vi "TEST - Trim Whitespace (Performance).vi"() -> ()   [LabVIEW 2009]
uses:
  source/library/Trim Whitespace/Trim Whitespace (String).vi
  source/library/Trim Whitespace 1/Trim Whitespace (String) 1.vi
panel:
  out "Time New (ms)":u32
  out "Time Old (ms)":u32
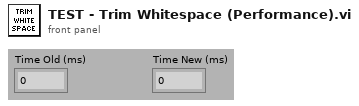
[diagram p1: front panel]
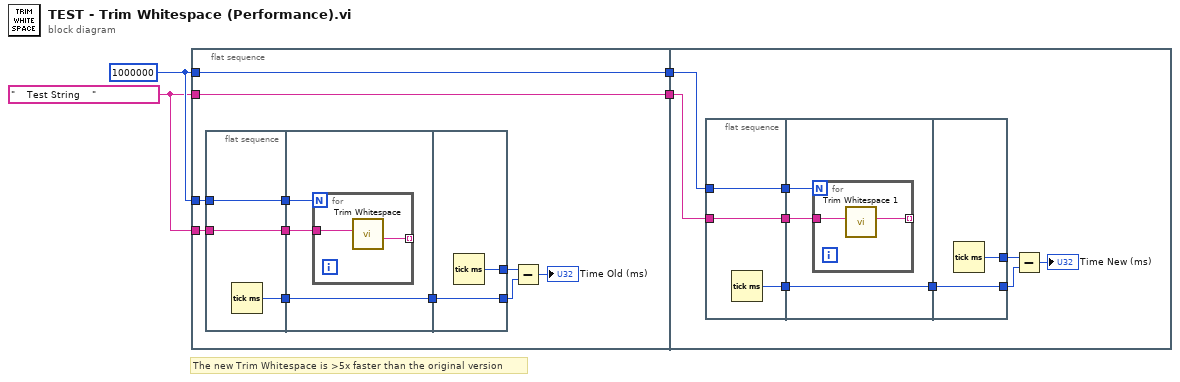
[diagram p0: block diagram]
diagram:
  w3 = 1000000
  w1 = "    Test String    " ("String in")
  # "The new Trim Whitespace is >5x faster than the original version"
  n1 = flat-sequence {
    tunnel: w3 -> [w8]
    tunnel: w1 -> [w7]
    tunnel: [w6] -> w4
    tunnel: w3 -> [w6]
    tunnel: [w5] -> w2
    tunnel: w1 -> [w5]
    tunnel: w4 -> [w27]
    tunnel: w2 -> [w26]
    frame #0 {
      n2 = flat-sequence {
        tunnel: [w18] -> w15
        tunnel: w7 -> [w17]
        tunnel: [w17] -> w14
        tunnel: [w16] -> w13
        tunnel: w8 -> [w16]
        tunnel: [w21] -> w12
        tunnel: w15 -> [w21]
        tunnel: w14 -> [w20]
        tunnel: w13 -> [w19]
        tunnel: [w25] -> w11
        tunnel: [w24] -> w10
        tunnel: w12 -> [w24]
        frame #0 {
          n3 = Tick Count (ms)() -> (millisecond timer value=w18:u32)
        }
        frame #1 {
          n4 = for {
            N: w19 -> [_]
            tunnel: w20 -> [w23]
            tunnel: [w22] -> _ mode=indexing
            n5 = call-poly "Trim Whitespace.vi"("String in"=w23) -> ("String out"=w22:string)  [unwired: 6 in]
          }
        }
        frame #2 {
          n6 = Tick Count (ms)() -> (millisecond timer value=w25:u32)
        }
      }
      n7 = Subtract(x=w11, y=w10) -> (x-y=→"Time Old (ms)":u32)
    }
    frame #1 {
      n8 = flat-sequence {
        tunnel: [w37] -> w34
        tunnel: [w35] -> w33
        tunnel: [w36] -> w32
        tunnel: w27 -> [w36]
        tunnel: w26 -> [w35]
        tunnel: [w40] -> w31
        tunnel: w34 -> [w40]
        tunnel: w33 -> [w39]
        tunnel: w32 -> [w38]
        tunnel: [w44] -> w30
        tunnel: [w43] -> w29
        tunnel: w31 -> [w43]
        frame #0 {
          n9 = Tick Count (ms)() -> (millisecond timer value=w37:u32)
        }
        frame #1 {
          n10 = for {
            N: w38 -> [_]
            tunnel: w39 -> [w42]
            tunnel: [w41] -> _ mode=indexing
            n11 = call-poly "Trim Whitespace 1.vi"("String in"=w42) -> ("String out"=w41:string)  [unwired: 8 in]
          }
        }
        frame #2 {
          n12 = Tick Count (ms)() -> (millisecond timer value=w44:u32)
        }
      }
      n13 = Subtract(x=w30, y=w29) -> (x-y=→"Time New (ms)":u32)
    }
  }
